vi "REFPROP1dll_Test.vi"(8 "error in (no error)":errorcluster) -> (0 "error out":errorcluster, 3 "Passed?":bool)   [LabVIEW 2021]
panel:
  out "Inputs":T1
  out "Outputs":T2
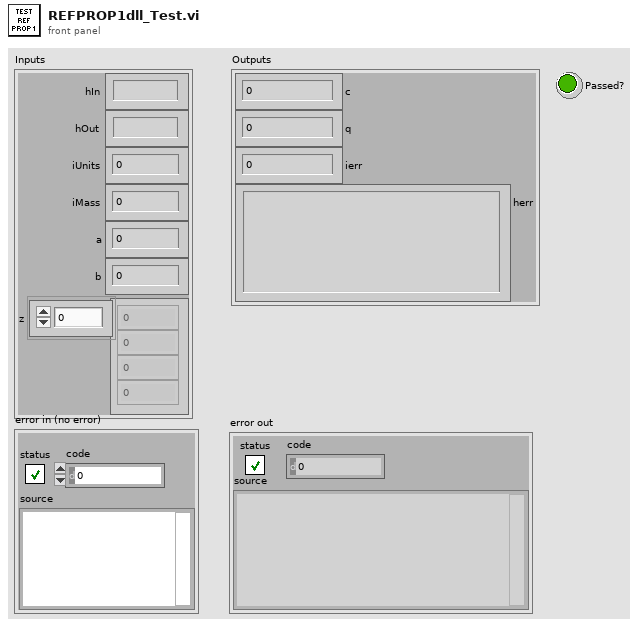
[diagram p1: front panel]
types:
  T1 = cluster{"hIn":string, "hOut":string, "iUnits":i32, "iMass":i32, "a":dbl, "b":dbl, "z":dbl[]}
  T2 = cluster{"c":dbl, "q":dbl, "ierr":i32, "herr":string}
  T3 = cluster{"hIn":string, "hOut":string, "iUnits":enum32{"DEFAULT", "MOLE SI", "MASS SI", "SI WITH C"}, "iMass":i32, "a":dbl, "b":dbl, "z":dbl[]}
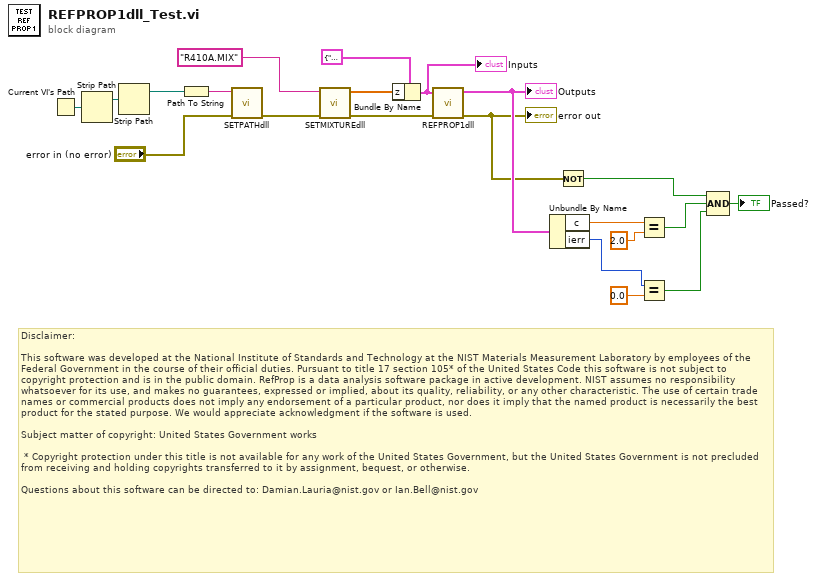
[diagram p0: block diagram]
diagram:
  # "Disclaimer:\n\nThis software was developed at the National Institute of Standards and Technology at the NIST Materials Measurement Laboratory by employees of the Federal Government in the course of their official duties. Pursuant to title 17 section 105* of the United States Code this software is not subject to copyright protection and is in the public domain. RefProp is a data analysis software package in active development. NIST assumes no responsibility whatsoever for its use, and makes no guarantees, expressed or implied, about its quality, reliability, or any other characteristic. The use of certain trade names or commercial products does not imply any endorsement of a particular product, nor does it imply that the named product is necessarily the best product for the stated purpose. We would appreciate acknowledgment if the software is used.\n \nSubject matter of copyright: United States Government works\n  \n * Copyright protection under this title is not available for any work of the United States Government, but the United States Government is not precluded from receiving and holding copyrights transferred to it by assignment, bequest, or otherwise.\n\nQuestions about this software can be directed to: Damian.Lauria@nist.gov or Ian.Bell@nist.gov"
  n1 = Current VI's Path() -> (path=w21:path)
  n2 = Strip Path(path=w21) -> (stripped path=w20:path)  [unwired: 1 out]
  n3 = Strip Path(path=w20) -> (stripped path=w19:path)  [unwired: 1 out]
  n4 = Path To String(path=w19) -> (string=w18:string)
  n5 = call "SETPATHdll.vi"("error in (no error)"="error in (no error)", "hpath"=w18) -> ("error out"=w17:errorcluster)  [unwired: 8 in, 1 out]
  n6 = call "SETMIXTUREdll.vi"("error in (no error)"=w17, "hmixnme"="R410A.MIX") -> ("error out"=w3:errorcluster, "z"=w16:dbl[])  [unwired: 7 in, 1 out]
  n7 = Bundle By Name(cluster=T3 {"hIn"="D", "hOut"="NCOMP", "iUnits"=enum."DEFAULT", "iMass"=0, "a"=313.5, "b"=632.0, "z"=[0.4, 0.6]} ("Inputs"), "z"=w16) -> (w15:T3)
  "Inputs" <- w15
  n8 = call "REFPROP1dll.vi"("error in (no error)"=w3, "Inputs"=w15) -> ("error out"=w2:errorcluster, "Outputs"=w11:T2)  [unwired: 8 in]
  "error out" <- w2
  "Outputs" <- w11
  n9 = Unbundle By Name(w11) -> ("c"=w10:dbl, "ierr"=w7:i32)
  n10 = Not(x=w2) -> (.not. x?=w12:bool)
  n11 = Equal?(x=w10, y=2.0 ("x")) -> (x = y?=w6:bool)
  n12 = Equal?(x=w7, y=0.0) -> (x = y?=w5:bool)
  n13 = Compound Arithmetic op=AND(w12, w6, w5) -> (→"Passed?":bool)
